vi "Timer.vi"(8 "PreMatchMetThisCycle?":dbl[](array[numeric]), 9 "PrimaryMetThisCycle?":dbl[](array[numeric]), 10 "Time Settings":T2, 11 "Run?":bool) -> (2 "Stopped":bool, 3 "Time Remaining":dbl, 4 "Unexpected Reset":bool, 5 "PrimaryMetThisCycle":bool[](array[boolean]), 6 "PreMatchMetThisCycle":bool[](array[boolean]), 7 "State":T1(ring)=enum."Pre-Primary")   [LabVIEW 2013]
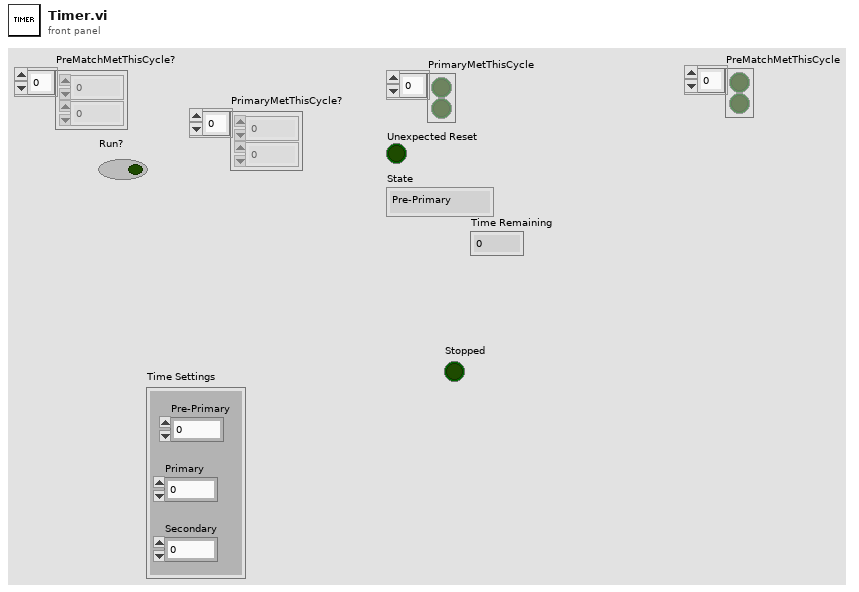
[diagram p1: front panel]
types:
  T1 = enum16{"Stopped", "Primary", "Secondary", "Pre-Primary"}
  T2 = cluster{"Primary":dbl, "Secondary":dbl, "Pre-Primary":dbl}
  T3 = enum16{"Get Timer State", "Start Timer", "Stop Timer"}
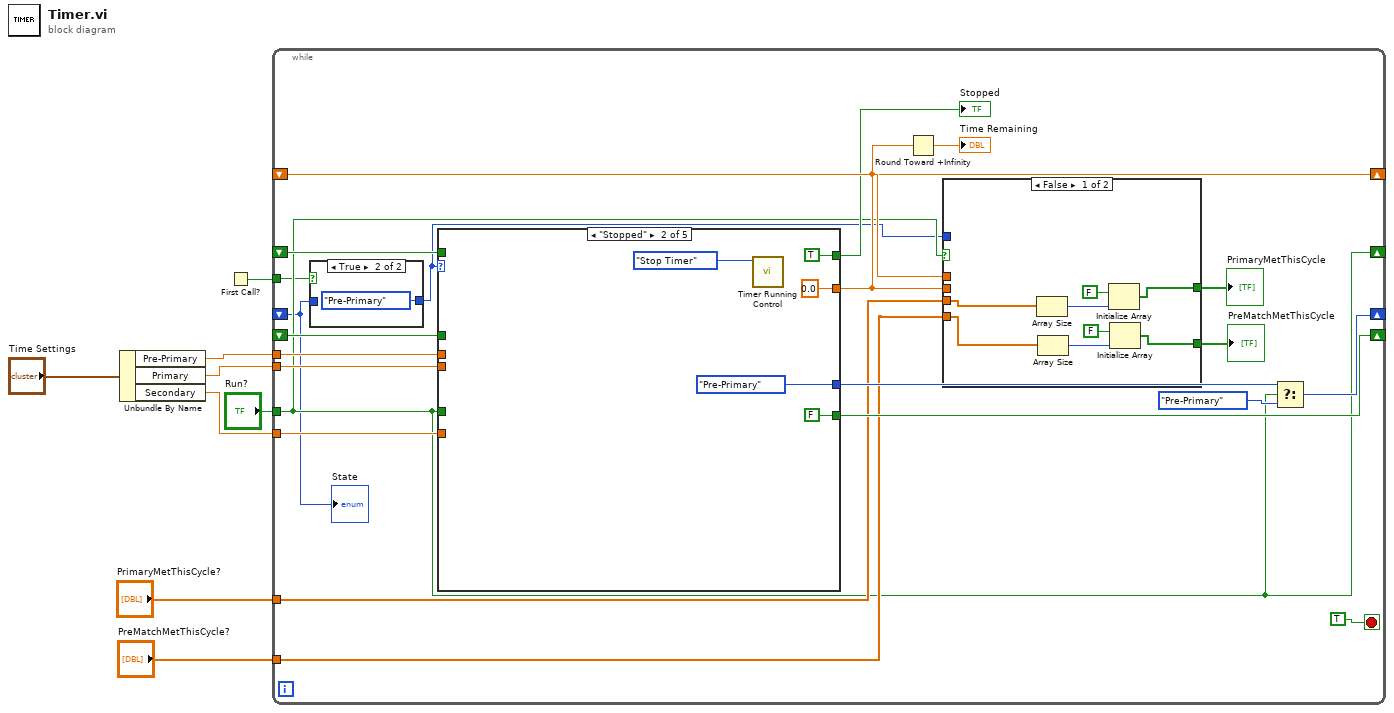
[diagram p0: block diagram]
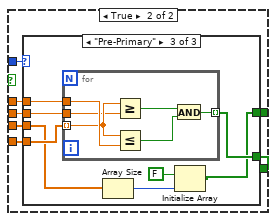
[diagram p3: hidden frame]
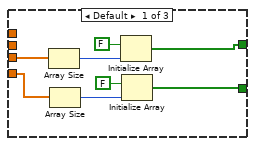
[diagram p4: hidden frame]
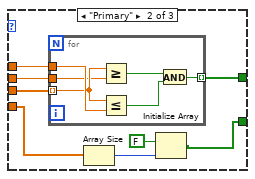
[diagram p5: hidden frame]
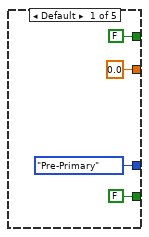
[diagram p6: hidden frame]
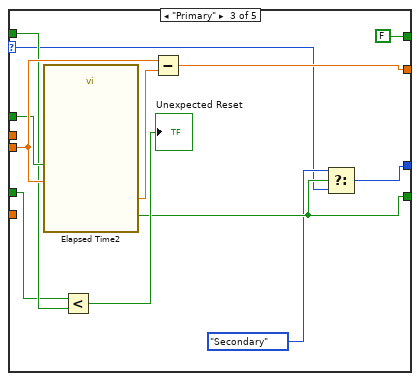
[diagram p7: hidden frame]
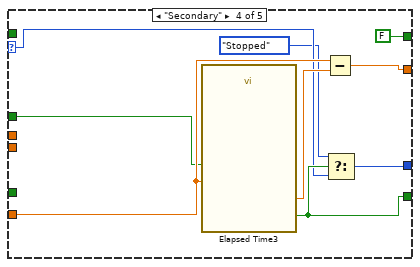
[diagram p8: hidden frame]
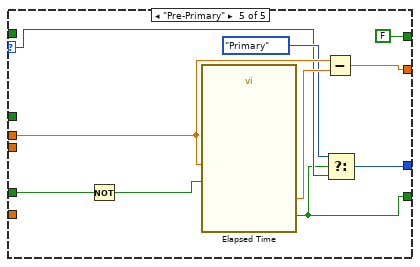
[diagram p9: hidden frame]
diagram:
  n1 = Unbundle By Name("Time Settings") -> ("Pre-Primary"=w4:dbl, "Primary"=w5:dbl, "Secondary"=w3:dbl)
  n2 = First Call?() -> (First Call?: T/F=w1:bool)
  n3 = while {
    tunnel: "Run?" -> [w13]
    tunnel: w5 -> [w28]
    tunnel: "PrimaryMetThisCycle?" -> [w21]
    shift-right: [w26] -> _
    shift-left: _ -> [w9]
    tunnel: w4 -> [w29]
    tunnel: w3 -> [w27]
    shift-right: [w13] -> _
    shift-left: _ -> [w17]
    shift-right: [w24] -> _
    shift-left: _ -> [w23]
    shift-right: [w18] -> _
    shift-left: _ -> [w20]
    tunnel: "PreMatchMetThisCycle?" -> [w15]
    tunnel: w1 -> [w11]
    stop <- TRUE stop-if-true
    n4 = case shown="True" w11 {
      tunnel: [w31 T1."Pre-Primary" ("f")] -> w10
      tunnel: w9 -> [w31 _]
      frame False {
      }
      frame True {
      }
    }
    n5 = case shown="\"Stopped\"" w10 {
      selector: w10 -> [_ _ w95 w108 w116]
      tunnel: w29 -> [_ _ _ _ w121]
      tunnel: w13 -> [_ _ w98 _ w122]
      tunnel: [0.0 0.0 w102 w111 w119] -> w18
      tunnel: [T1."Pre-Primary" ("State") T1."Pre-Primary" ("f") w94 w106 w117] -> w22
      tunnel: w28 -> [_ _ w104 _ _]
      tunnel: w27 -> [_ _ _ w113 _]
      tunnel: [FALSE ("Time has Elapsed") FALSE ("Time has Elapsed") w97 w109 w115] -> w24
      tunnel: w23 -> [_ _ w101 w110 _]
      tunnel: w17 -> [_ _ w100 _ _]
      tunnel: [FALSE TRUE FALSE FALSE FALSE] -> w14
      frame Default {
      }
      frame "Stopped" {
        n6 = call "Timer Running Control.vi"("Enum"=T3."Stop Timer") -> ()  [unwired: 10 in, 1 out]
      }
      frame "Primary" {
        n7 = call "Elapsed Time2"("Time Target (s)"=w104, "Reset"=w101) -> ("Elapsed Time (s)"=w103:dbl, "Time has Elapsed"=w97:bool)  [unwired: 10 in, 6 out]
        n8 = Less?(x=w98, y=w100) -> (x < y?=→"Unexpected Reset":bool)
        n9 = Subtract(x=w104, y=w103) -> (x-y=w102:dbl)
        n10 = Select(t=T1."Secondary" ("State"), s=w97, f=w95) -> (s? t:f=w94:T1)
      }
      frame "Secondary" {
        n11 = call "Elapsed Time3"("Time Target (s)"=w113, "Reset"=w110) -> ("Elapsed Time (s)"=w112:dbl, "Time has Elapsed"=w109:bool)  [unwired: 10 in, 6 out]
        n12 = Subtract(x=w113, y=w112) -> (x-y=w111:dbl)
        n13 = Select(t=T1."Stopped" ("State"), s=w109, f=w108) -> (s? t:f=w106:T1)
      }
      frame "Pre-Primary" {
        n14 = Not(x=w122) -> (.not. x?=w123:bool)
        n15 = call "Elapsed Time"("Time Target (s)"=w121, "Reset"=w123) -> ("Elapsed Time (s)"=w120:dbl, "Time has Elapsed"=w115:bool)  [unwired: 10 in, 6 out]
        n16 = Subtract(x=w121, y=w120) -> (x-y=w119:dbl)
        n17 = Select(t=T1."Primary" ("State"), s=w115, f=w116) -> (s? t:f=w117:T1)
      }
    }
    "Stopped" <- w14
    n18 = Round Toward +Infinity(x=w18) -> (ceil(x): smallest int >= x=→"Time Remaining":dbl)
    n19 = case shown="False" w13 {
      tunnel: w21 -> [w35 w47]
      tunnel: w20 -> [_ w46]
      tunnel: [w36 w45] -> w19
      tunnel: w10 -> [_ w44]
      tunnel: w18 -> [_ w43]
      tunnel: [w33 w42] -> w16
      tunnel: w15 -> [w34 w41]
      frame False {
        n20 = Array Size(array=w35) -> (size(s)=w40:i32)
        n21 = Array Size(array=w34) -> (size(s)=w37:i32)
        n22 = Initialize Array(FALSE, w40) -> (w36:bool[])
        n23 = Initialize Array(FALSE, w37) -> (w33:bool[])
      }
      frame True {
        n24 = case shown="\"Pre-Primary\"" w44 {
          tunnel: w47 -> [w55 w63 w70]
          tunnel: w43 -> [_ w61 w76]
          tunnel: w46 -> [_ w62 w77]
          tunnel: [w52 w60 w71] -> w45
          tunnel: [w48 w57 w75] -> w42
          tunnel: w41 -> [w49 w56 w74]
          frame Default {
            n25 = Array Size(array=w55) -> (size(s)=w54:i32)
            n26 = Array Size(array=w49) -> (size(s)=w50:i32)
            n27 = Initialize Array(FALSE, w54) -> (w52:bool[])
            n28 = Initialize Array(FALSE, w50) -> (w48:bool[])
          }
          frame "Primary" {
            n29 = for {
              tunnel: w63 -> [w68] mode=indexing
              tunnel: w62 -> [w69]
              tunnel: w61 -> [w67]
              tunnel: [w64] -> w60 mode=indexing
              n30 = Greater Or Equal?(x=w68, y=w67) -> (x >= y?=w66:bool)
              n31 = Less Or Equal?(x=w68, y=w69) -> (x <= y?=w65:bool)
              n32 = And(x=w66, y=w65) -> (x .and. y?=w64:bool)
            }
            n33 = Array Size(array=w56) -> (size(s)=w58:i32)
            n34 = Initialize Array(FALSE, w58) -> (w57:bool[])
          }
          frame "Pre-Primary" {
            n35 = for {
              tunnel: w74 -> [w82] mode=indexing
              tunnel: w77 -> [w83]
              tunnel: w76 -> [w81]
              tunnel: [w78] -> w75 mode=indexing
              n36 = Greater Or Equal?(x=w82, y=w81) -> (x >= y?=w80:bool)
              n37 = Less Or Equal?(x=w82, y=w83) -> (x <= y?=w79:bool)
              n38 = And(x=w80, y=w79) -> (x .and. y?=w78:bool)
            }
            n39 = Array Size(array=w70) -> (size(s)=w72:i32)
            n40 = Initialize Array(FALSE, w72) -> (w71:bool[])
          }
        }
      }
    }
    "PrimaryMetThisCycle" <- w19
    "PreMatchMetThisCycle" <- w16
    n41 = Select(t=w22, s=w13, f=T1."Pre-Primary") -> (s? t:f=w26:T1)
    "State" <- w9
  }
